vi "Process.vi"(8 "error in":errorcluster, 11 "LMT":refnum<class "LMT.lvclass">) -> (0 "error out":errorcluster, 3 "LMT out":refnum<class "LMT.lvclass">)   [LabVIEW 2017, in "LMT.lvclass"]
doc: "---------------------------------------------------------------\nJKI State Machine Objects™\nhttp://jki.net/state-machine-objects/\nCopyright (C) 2005-2015, JKI <info@jki.net>\nALL RIGHTS RESERVEDJKI State Machine Objects (SMO) 1.0.0.5\nJKI - JKI\nCopyright (c) 2016, JKI"
uses:
  LMT.lvclass
  D:/Program Files (x86)/National Instruments/LabVIEW 2017/vi.lib/JKI/JKI SMO/SMO/SMO.lvclass
  <vilib>/JKI/JKI SMO/SMO/Typedefs/SMOState --Enum.ctl
  <vilib>/JKI/JKI SMO/SMO/Typedefs/Parent Call--Enum.ctl
  <vilib>/JKI/JKI SMO/SMO/SMO.lvclass
panel:
  out "Dep2 GUID":string
  out "Dep1 GUID":string
  out "Dep2 Name":string
  out "Dep1 Name":string
  out "Dep2 State":T1
  out "Dep1 State":T1
  # "For instructions on how to use the JKI State Machine Objects, examples and video tutorials, visit:\nhttp://jki.net/state-machine-objects/\n\nJKI State Machine Objects™\nhttp://jki.net/state-machine-objects/\nCopyright (C) 2005-2015, JKI <info@jki.net>\nALL RIGHTS RESERVED"
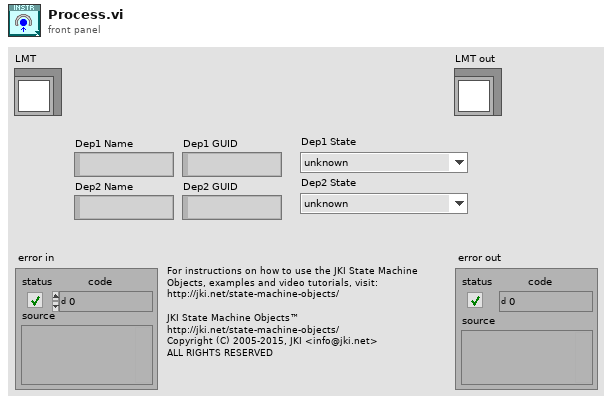
[diagram p1: front panel]
types:
  T1 = typedef "SMO.lvclass/SMOState --Enum.ctl" = enum16{"unknown", "Created", "Started", "Stopped"}
  T2 = typedef "SMO.lvclass/Parent Call--Enum.ctl" = enum16{"Allows parent to run", "Does not request parent to run"}
  T3 = enum32{"invalid app kind", "Development System", "Run Time System", "Student Edition", "Embedded LabVIEW", "Evaluation", "Custom"}
  T4 = enum32{"Invalid", "Standard", "Closed", "Hidden", "Minimized", "Maximized"}
  T5 = typedef "LMT.lvclass/Data.ctl" = string
  T6 = cluster{"Core":cluster{"Current VI Reference":refnum<vi>, "Close Panel on Exit?":bool, "error":errorcluster}, "Self Reference":refnum<class "LMT.lvclass">, "Your string data":string}
  T7 = cluster{"Current VI Reference":refnum<vi>, "Close Panel on Exit?":bool, "error":errorcluster}
  T8 = typedef "SMO.lvclass/Protected Events.ctl" = cluster{"StopProcesses":refnum<user-event>, "AbortProcesses":refnum<user-event>, "Config Changed":refnum<user-event>, "Dependency":refnum<user-event>}
  T9 = typedef "LMT.lvclass/ProtectedEvents--Cluster.ctl" = cluster{"API_Template":refnum<user-event>}
  T10 = typedef "LMT.lvclass/PrivateEvents--Cluster.ctl" = cluster{"AsyncMethod":refnum<user-event>}
  T11 = typedef "LMT.lvclass/Dependencies--Cluster.ctl" = cluster{"Dep1":refnum<class "SMO.lvclass">, "Dep2":refnum<class "SMO.lvclass">}
  T12 = typedef "SMO.lvclass/Public Events.ctl" = cluster{"Error":refnum<user-event>, "State":refnum<user-event>, "Reserve State":refnum<user-event>}
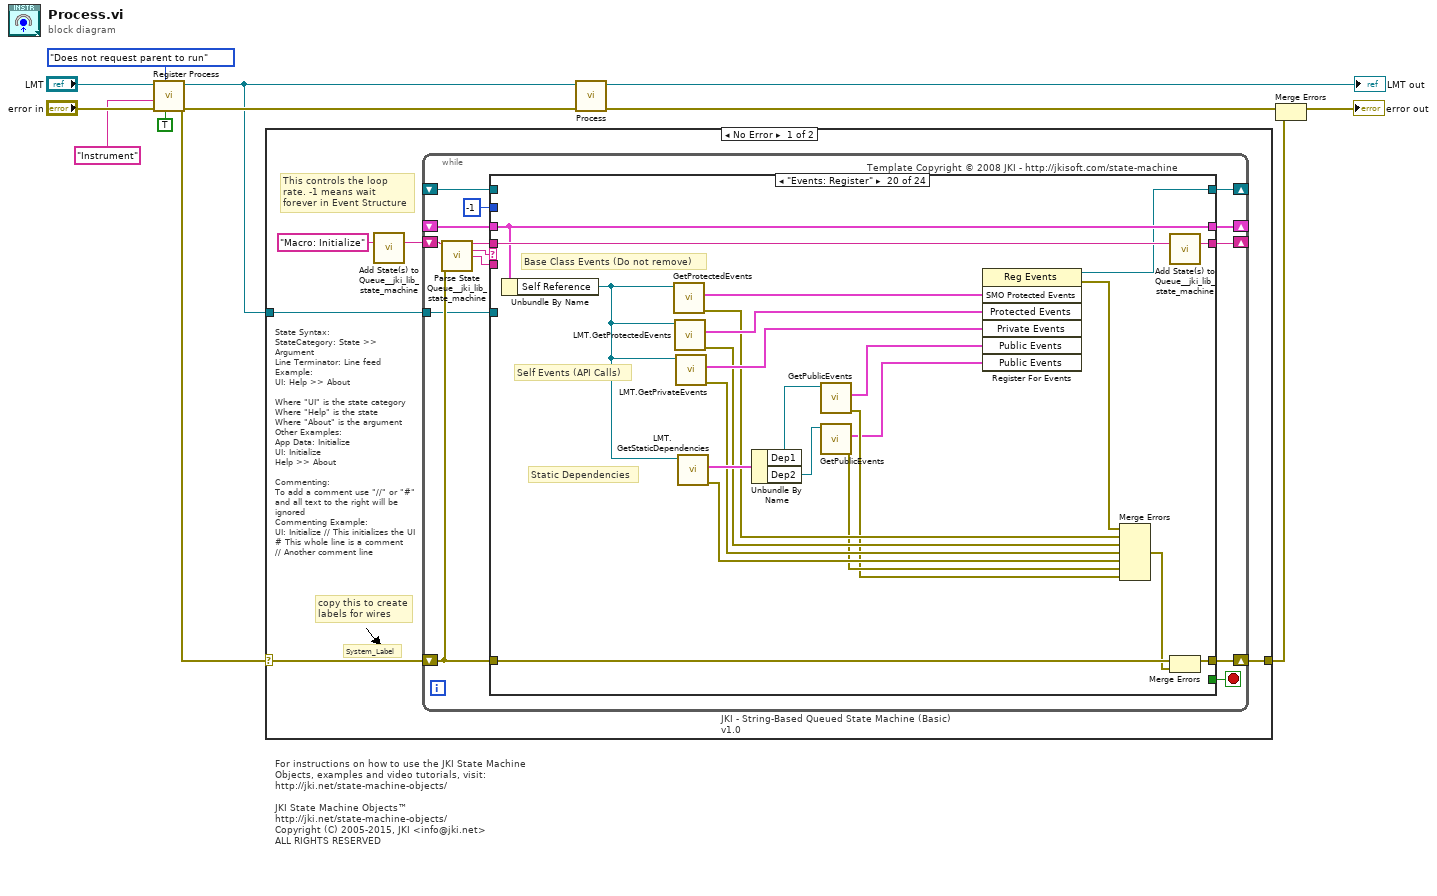
[diagram p0: block diagram]
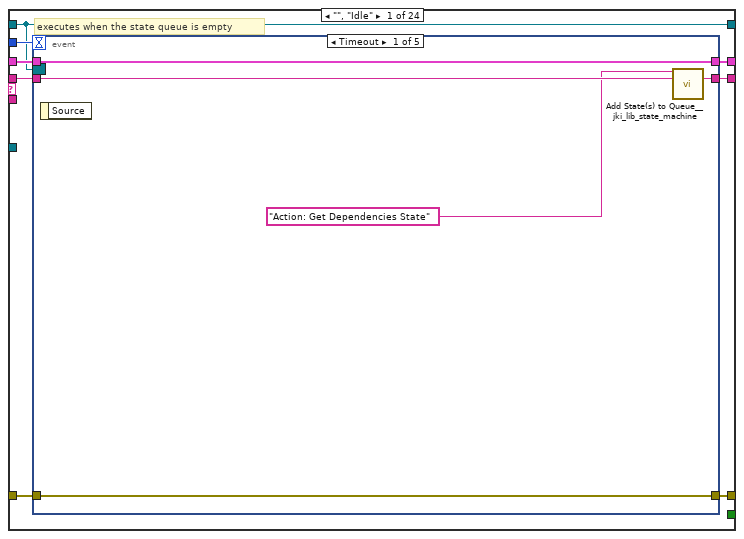
[diagram p2: hidden frame]
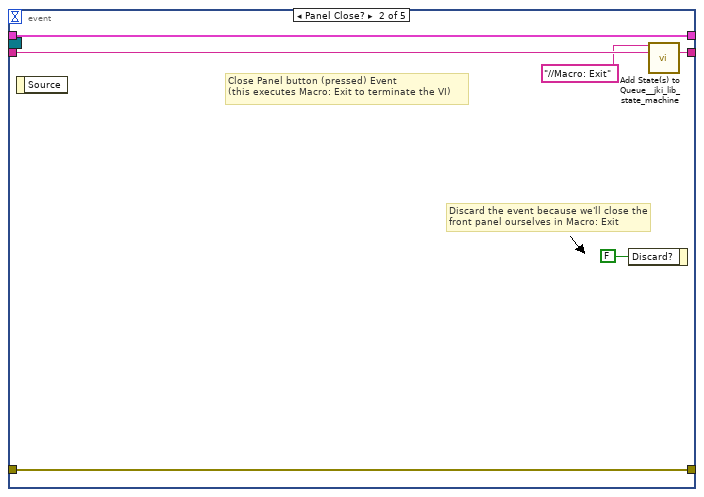
[diagram p3: hidden frame]
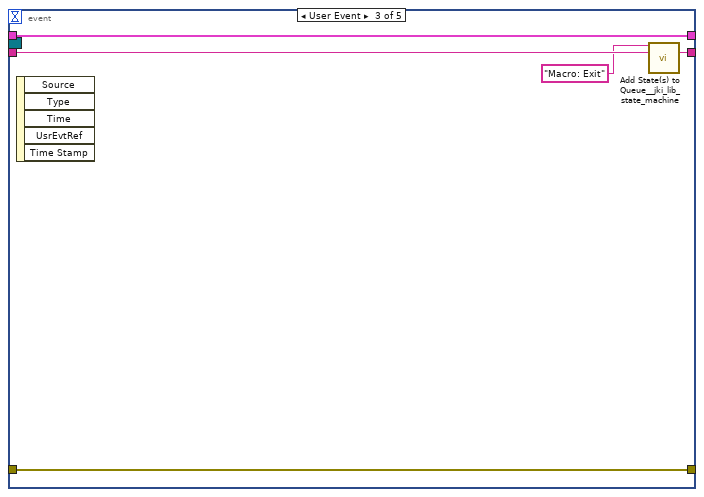
[diagram p4: hidden frame]
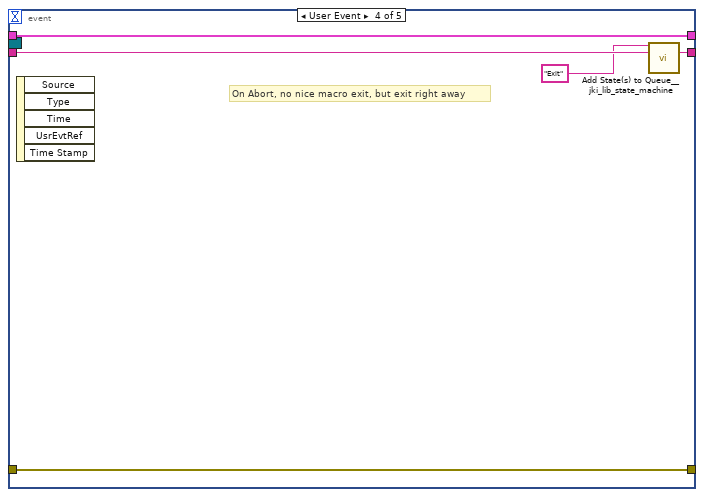
[diagram p5: hidden frame]
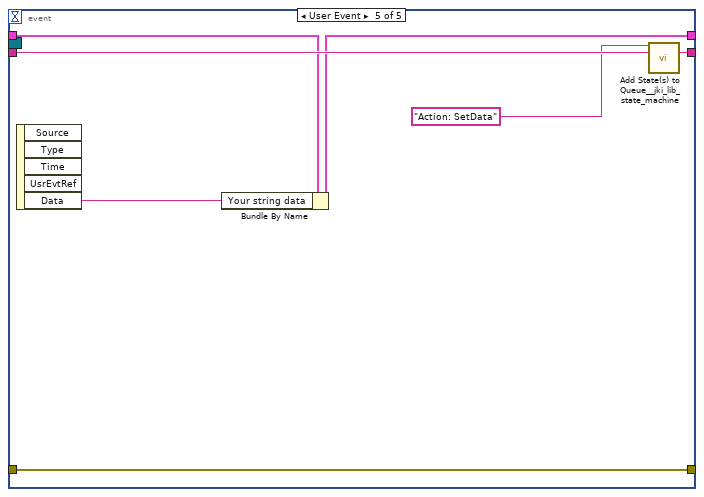
[diagram p6: hidden frame]
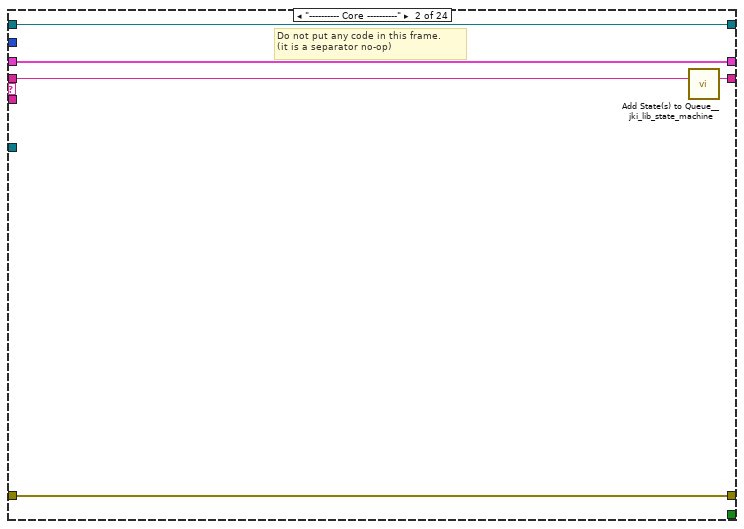
[diagram p7: hidden frame]
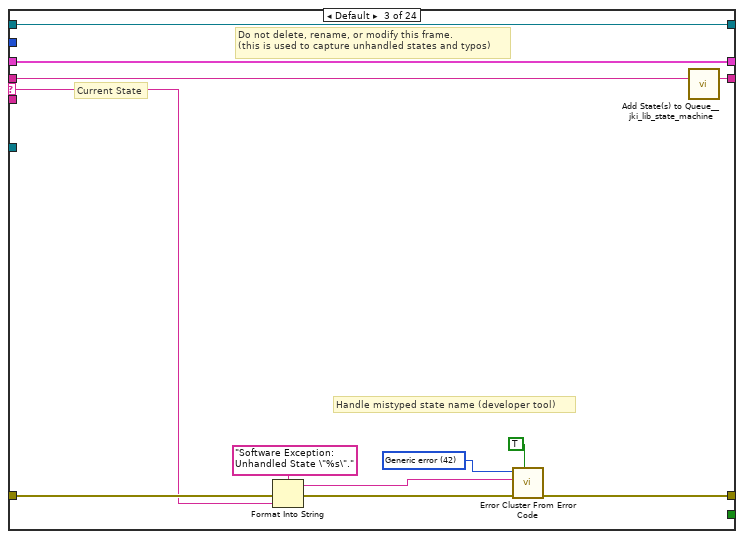
[diagram p8: hidden frame]
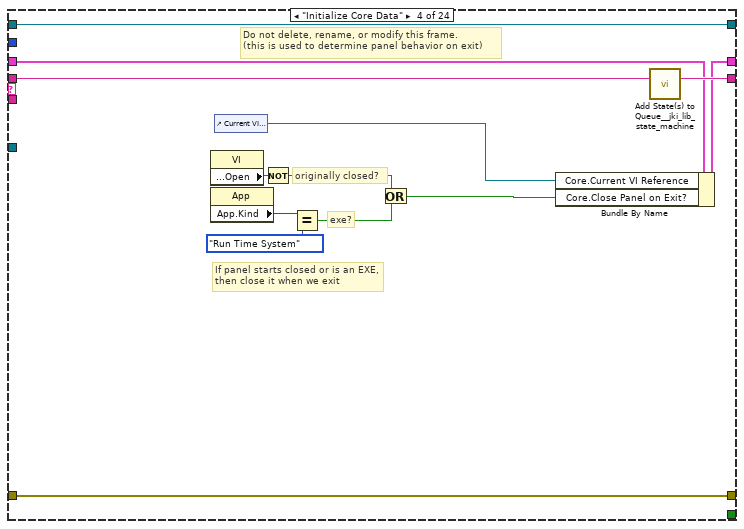
[diagram p9: hidden frame]
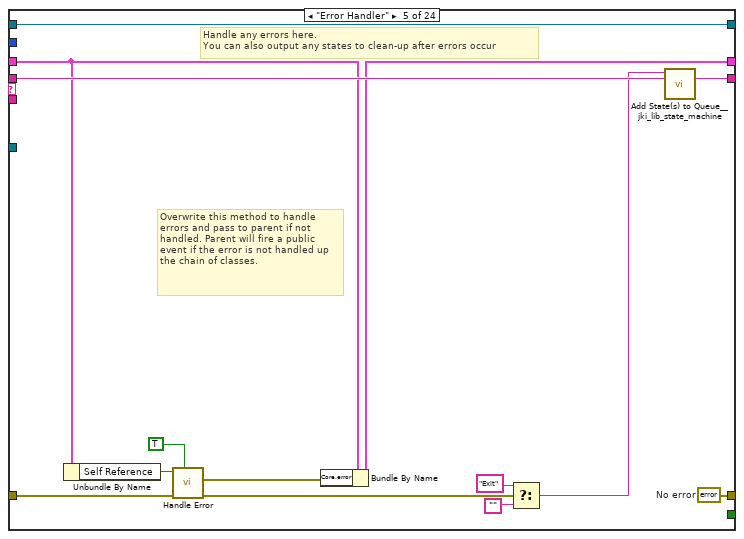
[diagram p10: hidden frame]
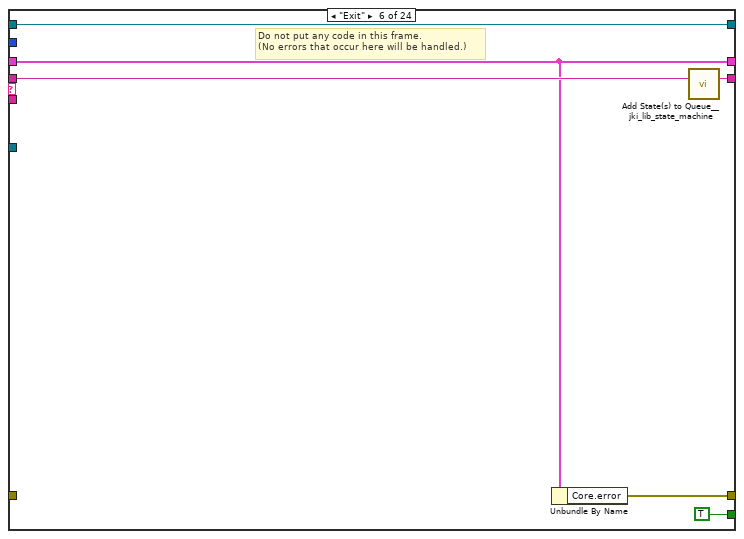
[diagram p11: hidden frame]
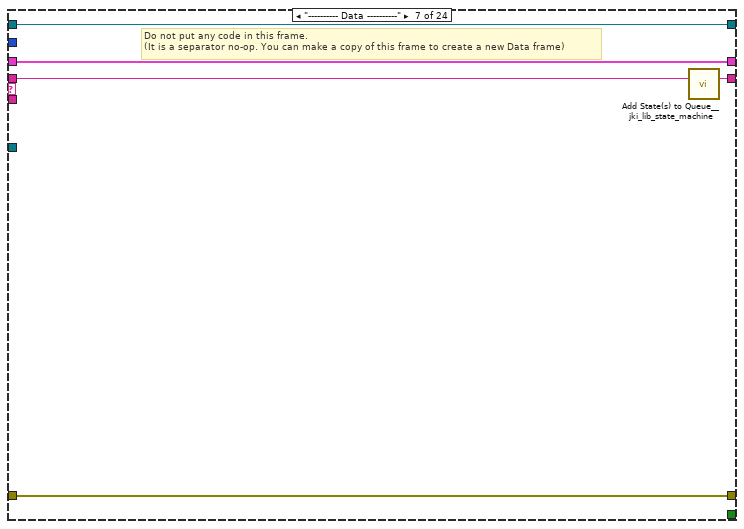
[diagram p12: hidden frame]
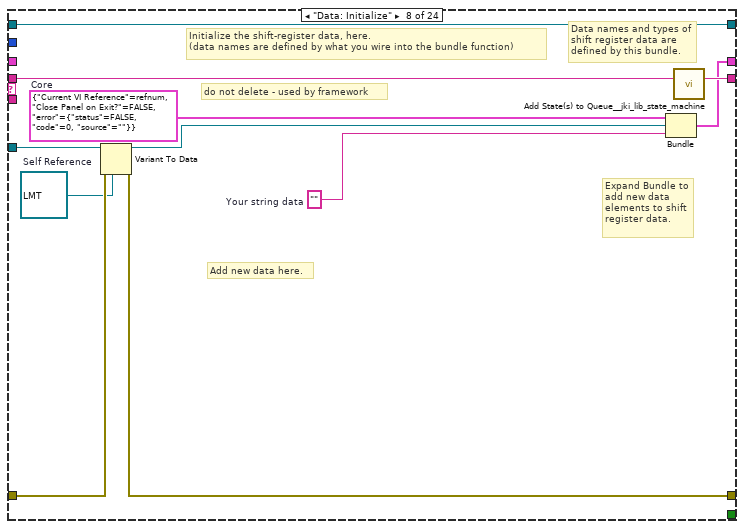
[diagram p13: hidden frame]
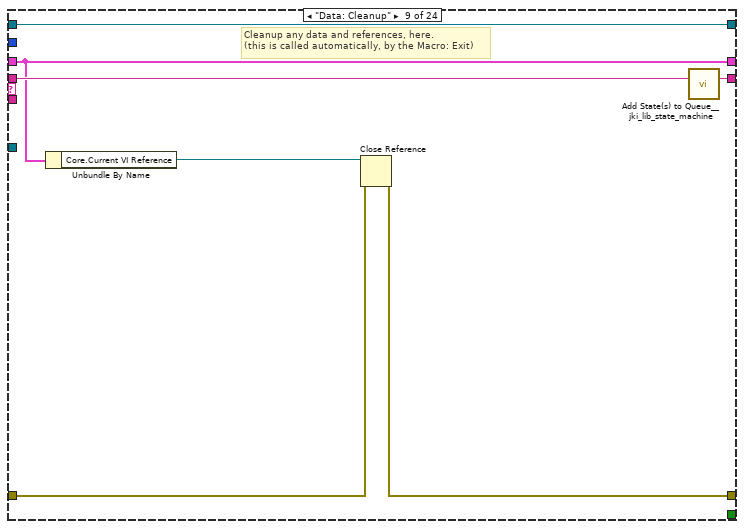
[diagram p14: hidden frame]
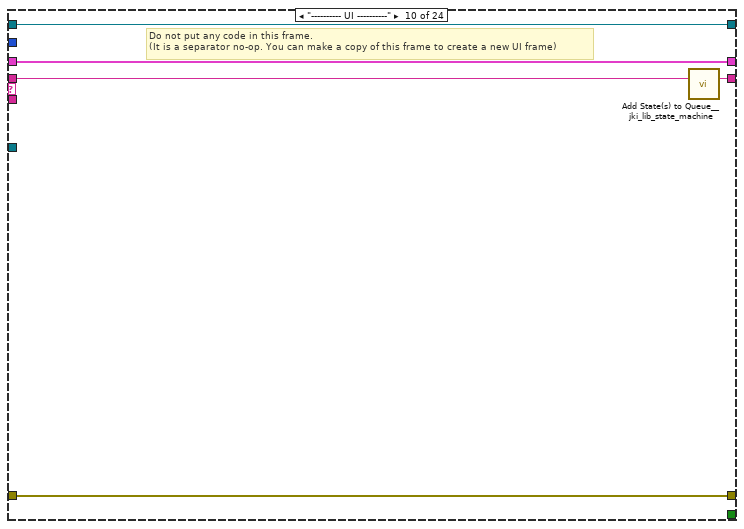
[diagram p15: hidden frame]
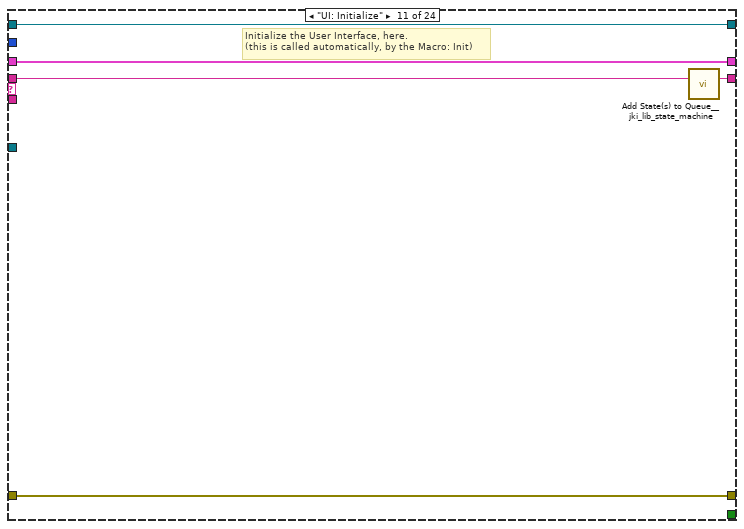
[diagram p16: hidden frame]
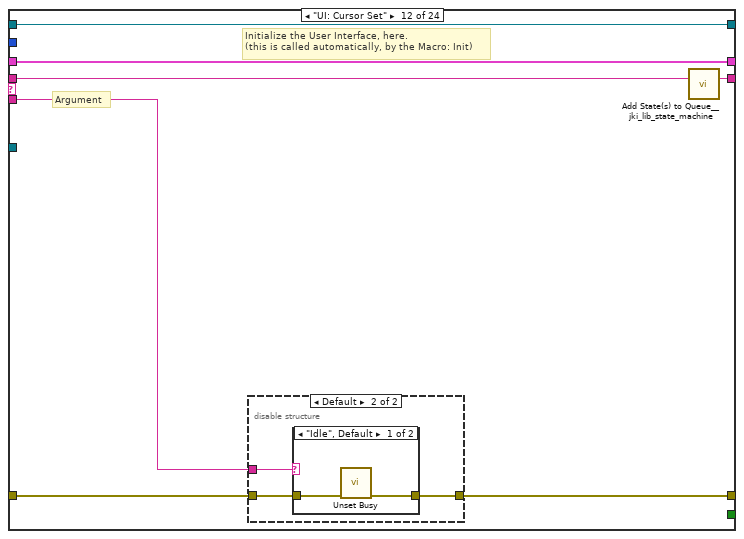
[diagram p17: hidden frame]
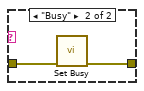
[diagram p19: hidden frame]
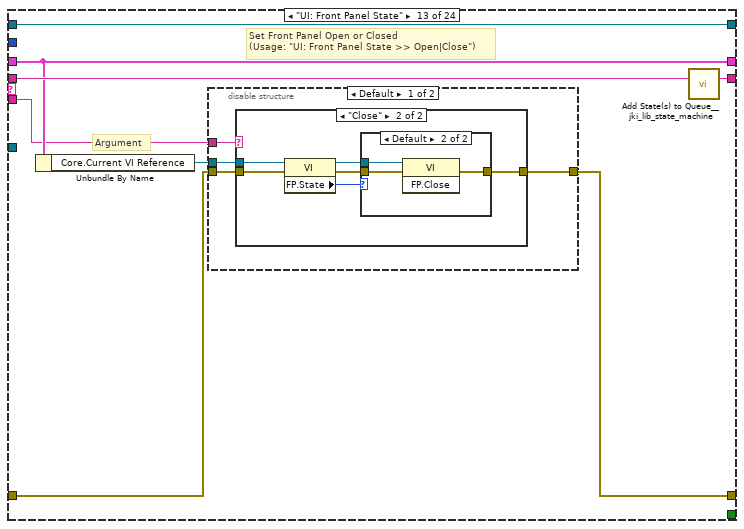
[diagram p20: hidden frame]
diagram:
  # "For instructions on how to use the JKI State Machine Objects, examples and video tutorials, visit:\nhttp://jki.net/state-machine-objects/\n\nJKI State Machine Objects™\nhttp://jki.net/state-machine-objects/\nCopyright (C) 2005-2015, JKI <info@jki.net>\nALL RIGHTS RESERVED"
  n1 = call <vilib>:"Register Process.vi"("Forces Self to Run (F)"=TRUE, "Parent Call"=Parent_Call--Enum."Does not request parent to run", "error in (no error)"="error in", "Process Name (optional)"="Instrument", "SMO"="LMT") -> ("error out"=w8:errorcluster, "SMO out"=w7:refnum<class "LMT.lvclass">)  [unwired: 5 in]
  n2 = case shown="No Error" w8 {
    selector: w8 -> [w13 w322]
    tunnel: w7 -> [w14 _]
    tunnel: [w12 w322] -> w4
    frame No Error {
      # "State Syntax:\nStateCategory: State >> Argument\nLine Terminator: Line feed\nExample:\nUI: Help >> About\n\nWhere \"UI\" is the state category\nWhere \"Help\" is the state\nWhere \"About\" is the argument\nOther Examples:\nApp Data: Initialize\nUI: Initialize\nHelp >> About\n\nCommenting:\nTo add a comment use \"//\" or \"#\" and all text to the right will be ignored\nCommenting Example:\nUI: Initialize // This initializes the UI\n# This whole line is a comment\n// Another comment line"
      # "copy this to create labels for wires"
      # "This controls the loop rate. -1 means wait forever in Event Structure"
      # "System_Label"
      n3 = call <vilib>:"Add State(s) to Queue__jki_lib_state_machine.vi"("State(s) in (\"\")"="Macro: Initialize") -> ("States Out"=w16:string)  [unwired: 14 in]
      n4 = while "JKI - String-Based Queued State Machine (Basic) v1.0" {
        shift-right: [w23] -> _
        shift-left: _ -> [w22]
        shift-right: [w26] -> w12
        shift-left: w13 -> [w20]
        shift-right: [w25] -> _
        shift-left: w16 -> [w27]
        tunnel: w14 -> [w19]
        shift-right: [w18] -> _
        shift-left: _ -> [w17]
        stop <- w24 stop-if-true
        # "Template Copyright © 2008 JKI - http://jkisoft.com/state-machine"
        n5 = call <vilib>:"Parse State Queue__jki_lib_state_machine.vi"("State Queue"=w27, "Error In (no error)"=w20) -> ("Remaining States"=w29:string, "Current State"=w30:string, "Arguments"=w28:string)  [unwired: 11 in]
        n6 = case shown="\"Events: Register\"" w30 {
          selector: w30 -> [_ _ w73 _ _ _ _ _ _ _ _ _ _ _ _ _ _ _ _ _ _ _ _ _]
          tunnel: w29 -> [w38 w71 w77 w96 w110 w116 w121 w132 w139 w144 w149 w156 w172 w204 w213 w227 w232 w243 w248 w271 w277 w282 w290 w318]
          tunnel: w28 -> [_ _ _ _ _ _ _ _ _ _ _ w150 w166 _ _ _ _ _ _ _ _ _ _ _]
          tunnel: w22 -> [w36 w68 w75 w87 w99 w112 w118 _ w134 w141 w147 w154 w168 w201 w209 w218 w229 w240 w245 w269 w275 w280 w287 w301]
          tunnel: [w35 w69 w79 w93 w101 w111 w119 w127 w135 w142 w146 w151 w169 w202 w211 w225 w230 w234 w246 w261 w273 w278 w283 w293] -> w26
          tunnel: w20 -> [w34 w69 w78 w93 w106 _ w119 w128 w136 w142 w146 w152 w170 w202 w211 w225 w230 w235 w246 w262 w273 w278 w284 w300]
          tunnel: [w37 w70 w76 w95 w109 w115 w120 w131 w138 w143 w148 w155 w171 w203 w212 w226 w231 w242 w247 w270 w276 w281 w289 w317] -> w25
          tunnel: [_ _ _ _ _ TRUE _ _ _ _ _ _ _ _ _ _ _ _ _ _ _ _ _ _] -> w24
          tunnel: [w33 w68 w75 w94 w98 w112 w118 w130 w134 w141 w147 w154 w168 w201 w209 w218 w229 w240 w245 w269 w275 w280 w287 w301] -> w23
          tunnel: -1 ("Timeout") -> [w32 _ _ _ _ _ _ _ _ _ _ _ _ _ _ _ _ _ _ _ _ _ _ _]
          tunnel: w19 -> [_ _ _ _ _ _ _ w125 _ _ _ _ _ _ _ _ _ _ _ _ _ _ _ _]
          tunnel: [w31 w67 w72 w84 w108 w113 w117 w123 w133 w140 w145 w153 w165 w200 w210 w219 w228 w241 w244 w268 w274 w279 w288 w316] -> w18
          tunnel: w17 -> [w31 w67 w72 w84 w108 w113 w117 w123 w133 w140 w145 w153 w165 w200 w210 w219 w228 w241 w244 _ w274 w279 w288 w316]
          frame "", "Idle" {
            # "executes when the state queue is empty"
            n7 = event shown="[0] Timeout" {
              selector: w31 -> [_ _ _ _ _]
              dyn-events: _ -> [_ _ _ _ _]
              timeout: w32 -> [_ _ _ _ _]
              tunnel: w38 -> [w43 w49 w54 w59 w66]
              tunnel: [w42 w48 w53 w58 w65] -> w37
              tunnel: w36 -> [w41 w46 w51 w56 w62]
              tunnel: [w40 w47 w52 w57 w64] -> w35
              tunnel: w34 -> [w40 w47 w52 w57 w64]
              tunnel: [w41 w46 w51 w56 w61] -> w33
              event Timeout {
                n8 = event-data() -> ()  [unwired: 1 in, 1 out]
                n9 = call <vilib>:"Add State(s) to Queue__jki_lib_state_machine.vi"("State(s) in Front (\"\")"="Action: Get Dependencies State", "State(s) in (\"\")"=w43) -> ("States Out"=w42:string)  [unwired: 13 in]
              }
              event Panel Close? {
                # "Discard the event because we'll close the front panel ourselves in Macro: Exit"
                # "Close Panel button (pressed) Event\n(this executes Macro: Exit to terminate the VI)"
                n10 = event-data() -> ()  [unwired: 1 in, 1 out]
                n11 = event-data("Discard?"=FALSE) -> ()  [unwired: 1 in, 1 out]
                n12 = call <vilib>:"Add State(s) to Queue__jki_lib_state_machine.vi"("State(s) in Front (\"\")"="//Macro: Exit", "State(s) in (\"\")"=w49) -> ("States Out"=w48:string)  [unwired: 13 in]
              }
              event User Event {
                n13 = event-data() -> ()  [unwired: 1 in, 5 out]
                n14 = call <vilib>:"Add State(s) to Queue__jki_lib_state_machine.vi"("State(s) in Front (\"\")"="Macro: Exit", "State(s) in (\"\")"=w54) -> ("States Out"=w53:string)  [unwired: 13 in]
              }
              event User Event {
                # "On Abort, no nice macro exit, but exit right away"
                n15 = event-data() -> ()  [unwired: 1 in, 5 out]
                n16 = call <vilib>:"Add State(s) to Queue__jki_lib_state_machine.vi"("State(s) in Front (\"\")"="Exit", "State(s) in (\"\")"=w59) -> ("States Out"=w58:string)  [unwired: 13 in]
              }
              event User Event {
                n17 = event-data() -> ("Data"=w63:T5)  [unwired: 1 in, 4 out]
                n18 = Bundle By Name(cluster=w62, "Your string data"=w63) -> (w61:T6)
                n19 = call <vilib>:"Add State(s) to Queue__jki_lib_state_machine.vi"("State(s) in Front (\"\")"="Action: SetData", "State(s) in (\"\")"=w66) -> ("States Out"=w65:string)  [unwired: 13 in]
              }
            }
          }
          frame "---------- Core ----------" {
            # "Do not put any code in this frame.\n(it is a separator no-op)"
            n20 = call <vilib>:"Add State(s) to Queue__jki_lib_state_machine.vi"("State(s) in (\"\")"=w71) -> ("States Out"=w70:string)  [unwired: 14 in]
          }
          frame Default {
            w82 = 42 items=["No error", "Argument error", "Memory is full", "Out of zone", "End of file", "File already open", "Generic file I/O error", "File not found", "File permission error", "Disk is full", "Duplicate path", "Too many files open", "System feature not enabled", "Resource file not found", "Cannot add resource", "Resource not found", "Image not found", "Image memory error", "Pen does not exist", "Config type invalid", "Config token not found", "Config parse error", "Config memory error", "Bad external code format", "Bad external code offset", "External code not present", "Null window", "Destroy window error", "Null menu", "Print aborted", "Bad print record", "Print driver error", "Windows error during printing", "Memory error during printing", "Print dialog error", "Generic print error", "Invalid device refnum", "Device not found", "Device parameter error", "Device unit error", "Cannot open device", "Device call aborted", "Generic error", "Cancelled by user", "Object ID too low", "Object ID too high", "Object not in heap", "Unknown heap", "Unknown object (invalid DefProc)", "Unknown object (DefProc not in table)", "Message out of range", "Invalid (null) method", "Unknown message", "Manager call not supported", "Bad address", "Network operation in progress", "Network operation timed out", "Connection is busy", "Network attribute not supported", "Network error", "Address in use", "System out of memory", "Connection aborted", "Connection refused", "Not connected", "Already connected", "Connection closed", "Initialization error (interapplication manager)", "Bad occurrence", "Wait on unbound occurrence handler", "Occurrence queue overflow", "Datalog type conflict", "Unused", "Unrecognized type (interapplication manager)", "Memory corrupt", "Failed to make temporary DLL", "Old CIN version", "Drag socket not found", "Failed to load drop-object", "Failed to register OLE object", "Failed to release OLE object", "Format specifier type mismatch", "Unknown format specifier", "Too few format specifiers", "Too many format specifiers", "Scan failed", "Newer CIN version", "Error converting to variant", "Runtime menu error", "Password tampered", "Variant attribute not found", "Incompatible variant data type", "Event data is not available", "Event Store is not present", "Occurrence is not found", "Event Queue is not created", "Event info is not available", "Refnum passed is NULL", "Error retrieving Class GUID", "Error retrieving CoClass GUID", "Error retrieving TypeLib GUID.", "Bad built application magic bytes.", "Specific driver is different from the specific driver associated with the Logical Name.", "There is no session opened to the class driver.", "Max Error", "MAX - Error with config objects", "MAX - Error loading configuration", "MAX - Group not supported"]
            # "Current State"
            # "Do not delete, rename, or modify this frame.\n(this is used to capture unhandled states and typos)"
            # "Handle mistyped state name (developer tool)"
            n21 = Format Into String(format string="Software Exception: Unhandled State \"%s\"." ("message"), error in=w78, w73) -> (resulting string=w81:string, error out=w80:errorcluster)  [unwired: 1 in]
            n22 = call <vilib>:"Error Cluster From Error Code.vi"("show call chain? (False)"=TRUE, "error in (no error)"=w80, "error message (\"\")"=w81, "error code (0)"=w82) -> ("error out"=w79:errorcluster)  [unwired: 5 in]
            n23 = call <vilib>:"Add State(s) to Queue__jki_lib_state_machine.vi"("State(s) in (\"\")"=w77) -> ("States Out"=w76:string)  [unwired: 14 in]
          }
          frame "Initialize Core Data" {
            # "Do not delete, rename, or modify this frame.\n(this is used to determine panel behavior on exit)"
            # "originally closed?"
            # "exe?"
            # "If panel starts closed or is an EXE, then close it when we exit"
            n24 = property class="VI"() -> ("Front Panel.Open"=w92:bool)  [unwired: 2 in, 2 out]
            n25 = property class="App"() -> ("App.Kind"=w91:T3)  [unwired: 2 in, 2 out]
            n26 = control-ref of="Current VI Reference"() -> (w85:refnum<vi>)
            n27 = Not(x=w92) -> (.not. x?=w89:bool)
            n28 = Equal?(x=w91, y=T3."Run Time System" ("Application:Kind")) -> (x = y?=w88:bool)
            n29 = Or(x=w89, y=w88) -> (x .or. y?=w86:bool)
            n30 = Bundle By Name(cluster=w87, "Core.Current VI Reference"=w85, "Core.Close Panel on Exit?"=w86) -> (w94:T6)
            n31 = call <vilib>:"Add State(s) to Queue__jki_lib_state_machine.vi"("State(s) in (\"\")"=w96) -> ("States Out"=w95:string)  [unwired: 14 in]
          }
          frame "Error Handler" {
            w101 = errorcluster {"status"=FALSE, "code"=0, "source"=""}  # No error
            # "Overwrite this method to handle errors and pass to parent if not handled. Parent will fire a public event if the error is not handled up the chain of classes."
            # "Handle any errors here.\nYou can also output any states to clean-up after errors occur"
            n32 = Unbundle By Name(w99) -> ("Self Reference"=w107:refnum<class "LMT.lvclass">)
            n33 = call-dynamic "Handle Error.vi"("Stop on Unhandled Error (T)"=TRUE, "error in"=w106, "SMO"=w107) -> ("handling error"=w102:errorcluster, "Unhandled error"=w100:errorcluster)  [unwired: 6 in, 1 out]
            n34 = Bundle By Name(cluster=w99, "Core.error"=w100) -> (w98:T6)
            n35 = Select(t="Exit", s=w102, f="") -> (s? t:f=w103:string)
            n36 = call <vilib>:"Add State(s) to Queue__jki_lib_state_machine.vi"("State(s) in Front (\"\")"=w103, "State(s) in (\"\")"=w110) -> ("States Out"=w109:string)  [unwired: 13 in]
          }
          frame "Exit" {
            # "Do not put any code in this frame.\n(No errors that occur here will be handled.)"
            n37 = Unbundle By Name(w112) -> ("Core.error"=w111:errorcluster)
            n38 = call <vilib>:"Add State(s) to Queue__jki_lib_state_machine.vi"("State(s) in (\"\")"=w116) -> ("States Out"=w115:string)  [unwired: 14 in]
          }
          frame "---------- Data ----------" {
            # "Do not put any code in this frame.\n(It is a separator no-op. You can make a copy of this frame to create a new Data frame)"
            n39 = call <vilib>:"Add State(s) to Queue__jki_lib_state_machine.vi"("State(s) in (\"\")"=w121) -> ("States Out"=w120:string)  [unwired: 14 in]
          }
          frame "Data: Initialize" {
            w122 = T7 {"Current VI Reference"=refnum, "Close Panel on Exit?"=FALSE, "error"={"status"=FALSE, "code"=0, "source"=""}}  # Core
            w126 = refnum<class "LMT.lvclass"> refnum  # Self Reference
            w129 = ""  # Your string data
            # "do not delete - used by framework"
            # "Expand Bundle to add new data elements to shift register data."
            # "Add new data here."
            # "Data names and types of shift register data are defined by this bundle."
            # "Initialize the shift-register data, here.\n(data names are defined by what you wire into the bundle function)"
            n40 = Variant To Data(error in=w128, type=w126, Variant=w125) -> (data=w124:refnum<class "LMT.lvclass">, error out=w127:errorcluster)
            n41 = Bundle("Core"=w122, "Self Reference"=w124, "Your string data"=w129) -> (w130:T6)  [unwired: 1 in]
            n42 = call <vilib>:"Add State(s) to Queue__jki_lib_state_machine.vi"("State(s) in (\"\")"=w132) -> ("States Out"=w131:string)  [unwired: 14 in]
          }
          frame "Data: Cleanup" {
            # "Cleanup any data and references, here.\n(this is called automatically, by the Macro: Exit)"
            n43 = Unbundle By Name(w134) -> ("Core.Current VI Reference"=w137:refnum<vi>)
            n44 = Close Reference(reference=w137, error in (no error)=w136) -> (error out=w135:errorcluster)
            n45 = call <vilib>:"Add State(s) to Queue__jki_lib_state_machine.vi"("State(s) in (\"\")"=w139) -> ("States Out"=w138:string)  [unwired: 14 in]
          }
          frame "---------- UI ----------" {
            # "Do not put any code in this frame.\n(It is a separator no-op. You can make a copy of this frame to create a new UI frame)"
            n46 = call <vilib>:"Add State(s) to Queue__jki_lib_state_machine.vi"("State(s) in (\"\")"=w144) -> ("States Out"=w143:string)  [unwired: 14 in]
          }
          frame "UI: Initialize" {
            # "Initialize the User Interface, here.\n(this is called automatically, by the Macro: Init)"
            n47 = call <vilib>:"Add State(s) to Queue__jki_lib_state_machine.vi"("State(s) in (\"\")"=w149) -> ("States Out"=w148:string)  [unwired: 14 in]
          }
          frame "UI: Cursor Set" {
            # "Argument"
            # "Initialize the User Interface, here.\n(this is called automatically, by the Macro: Init)"
            n48 = disable-structure shown="Default" {
              disable-tunnel: w152 -> [w157 w160]
              disable-tunnel: [w157 w159] -> w151
              disable-tunnel: w150 -> [_ w158]
              frame condition #0 {
              }
              frame condition #1 (active) {
                n49 = case shown="\"Idle\", Default" w158 {
                  tunnel: w160 -> [w162 w164]
                  tunnel: [w161 w163] -> w159
                  frame "Idle", Default {
                    n50 = call <vilib>:"Unset Busy.vi"("error in (no error)"=w162) -> ("error out"=w161:errorcluster)  [unwired: 10 in]
                  }
                  frame "Busy" {
                    n51 = call <vilib>:"Set Busy.vi"("error in (no error)"=w164) -> ("error out"=w163:errorcluster)  [unwired: 9 in, 1 out]
                  }
                }
              }
            }
            n52 = call <vilib>:"Add State(s) to Queue__jki_lib_state_machine.vi"("State(s) in (\"\")"=w156) -> ("States Out"=w155:string)  [unwired: 14 in]
          }
          frame "UI: Front Panel State" {
            # "Argument"
            # "Set Front Panel Open or Closed\n(Usage: \"UI: Front Panel State >> Open|Close\")"
            n53 = Unbundle By Name(w168) -> ("Core.Current VI Reference"=w167:refnum<vi>)
            n54 = disable-structure shown="Default" {
              disable-tunnel: w170 -> [w176 w199]
              disable-tunnel: [w175 w199] -> w169
              disable-tunnel: w167 -> [w174 _]
              disable-tunnel: w166 -> [w173 _]
              frame condition #0 (active) {
                n55 = case shown="\"Close\"" w173 {
                  tunnel: w176 -> [w180 w193]
                  tunnel: [w182 w194] -> w175
                  tunnel: w174 -> [w181 w191]
                  frame "Open", Default {
                    n56 = property class="VI"(reference=w181, error in=w180) -> (reference out=w178:refnum<vi>, error out=w179:errorcluster, "FP.State"=w177:T4)
                    n57 = case shown="\"Closed\"" w177 {
                      tunnel: [w185 w188] -> w182
                      tunnel: w179 -> [w184 w188]
                      tunnel: w178 -> [w183 _]
                      frame "Closed" {
                        n58 = invoke class="VI" method="FP.Open"(reference=w183, error in=w184, "Activate"=TRUE, "State"=T4."Standard") -> (error out=w185:errorcluster)  [unwired: 1 in, 4 out]
                      }
                      frame Default {
                      }
                    }
                  }
                  frame "Close" {
                    n59 = property class="VI"(reference=w191, error in=w193) -> (reference out=w190:refnum<vi>, error out=w192:errorcluster, "FP.State"=w189:T4)
                    n60 = case shown="Default" w189 {
                      tunnel: [w195 w198] -> w194
                      tunnel: w192 -> [w195 w197]
                      tunnel: w190 -> [_ w196]
                      frame "Invalid", "Closed" {
                      }
                      frame Default {
                        n61 = invoke class="VI" method="FP.Close"(reference=w196, error in=w197) -> (error out=w198:errorcluster)  [unwired: 1 in, 2 out]
                      }
                    }
                  }
                }
              }
              frame condition #1 {
              }
            }
            n62 = call <vilib>:"Add State(s) to Queue__jki_lib_state_machine.vi"("State(s) in (\"\")"=w172) -> ("States Out"=w171:string)  [unwired: 14 in]
          }
          frame "---------- Macro ----------" {
            # "Do not put any code in this frame.\n(It is a separator no-op. You can make a copy of this frame to create a new Macro frame)"
            n63 = call <vilib>:"Add State(s) to Queue__jki_lib_state_machine.vi"("State(s) in (\"\")"=w204) -> ("States Out"=w203:string)  [unwired: 14 in]
          }
          frame "Macro: Initialize" {
            w207 = "UI: Initialize\n//UI: Front Panel State >> Open"  # UI: Initialize //UI: Front Panel State >> Open
            # "Initialization Macro\n(This is called once, when the VI starts)"
            n64 = call <vilib>:"Add State(s) to Queue__jki_lib_state_machine.vi"("State(s) in Front (\"\")"="Data: Initialize\nInitialize Core Data\nEvents: Register\nAction: Get Dependencies State", "State(s) in (\"\")"="Process: Sync", "State(s) at Back (\"\")"=w207) -> ("States Out"=w206:string)  [unwired: 12 in]
            n65 = call <vilib>:"Add State(s) to Queue__jki_lib_state_machine.vi"("State(s) in Front (\"\")"=w206, "State(s) in (\"\")"=w213) -> ("States Out"=w212:string)  [unwired: 13 in]
          }
          frame "Macro: Exit" {
            # "Exit Macro\n(This is called once, when the VI exits)"
            n66 = Unbundle By Name(w218) -> ("Core.Close Panel on Exit?"=w224:bool)
            n67 = Select(t="UI: Front Panel State >> Close", s=w224, f="") -> (s? t:f=w221:string)
            n68 = call <vilib>:"Add State(s) to Queue__jki_lib_state_machine.vi"("State(s) in Front (\"\")"="Data: Cleanup\nEvents: Unregister", "State(s) in (\"\")"="Process: Sync", "State(s) at Back (\"\")"="Action: Get Dependencies State\nExit") -> ("States Out"=w215:string)  [unwired: 12 in]
            n69 = call <vilib>:"Add State(s) to Queue__jki_lib_state_machine.vi"("State(s) in (\"\")"=w221, "State(s) at Back (\"\")"=w215) -> ("States Out"=w220:string)  [unwired: 13 in]
            n70 = call <vilib>:"Add State(s) to Queue__jki_lib_state_machine.vi"("State(s) in Front (\"\")"=w220, "State(s) in (\"\")"=w227) -> ("States Out"=w226:string)  [unwired: 13 in]
          }
          frame "---------- Process ----------" {
            # "Template Separator\n(You can make a copy of, or modify, this frame)"
            n71 = call <vilib>:"Add State(s) to Queue__jki_lib_state_machine.vi"("State(s) in (\"\")"=w232) -> ("States Out"=w231:string)  [unwired: 14 in]
          }
          frame "Process: Sync" {
            n72 = Unbundle By Name(w240) -> ("Self Reference"=w236:refnum<class "LMT.lvclass">)
            n73 = call <vilib>:"WaitOnProcessSync.vi"("error in (no error)"=w235, "SMO"=w236) -> ("error out"=w234:errorcluster, "Don't run?"=w239:bool)  [unwired: 7 in, 1 out]
            n74 = Select(t="Data: Cleanup\nEvents: Unregister\nExit", s=w239, f="") -> (s? t:f=w233:string)
            n75 = call <vilib>:"Add State(s) to Queue__jki_lib_state_machine.vi"("State(s) in Front (\"\")"=w233, "State(s) in (\"\")"=w243) -> ("States Out"=w242:string)  [unwired: 13 in]
          }
          frame "---------- Events ----------" {
            # "Template Separator\n(You can make a copy of, or modify, this frame)"
            n76 = call <vilib>:"Add State(s) to Queue__jki_lib_state_machine.vi"("State(s) in (\"\")"=w248) -> ("States Out"=w247:string)  [unwired: 14 in]
          }
          frame "Events: Register" {
            # "Static Dependencies"
            # "Self Events (API Calls)"
            # "Base Class Events (Do not remove)"
            n77 = Unbundle By Name(w269) -> ("Self Reference"=w264:refnum<class "LMT.lvclass">)
            n78 = call <vilib>:"GetProtectedEvents.vi"("SMO"=w264) -> ("error out"=w259:errorcluster, "SMO Protected Events"=w267:T8)  [unwired: 8 in, 1 out]
            n79 = call "LMT.GetProtectedEvents.vi"("LMT"=w264) -> ("error out"=w258:errorcluster, "Protected Events"=w266:T9)  [unwired: 8 in, 1 out]
            n80 = call "LMT.GetPrivateEvents.vi"("LMT"=w264) -> ("error out"=w257:errorcluster, "Private Events"=w265:T10)  [unwired: 8 in, 1 out]
            n81 = call "LMT.GetStaticDependencies.vi"("LMT"=w264) -> ("error out"=w256:errorcluster, "Dependencies"=w263:T11)  [unwired: 8 in, 1 out]
            n82 = Unbundle By Name(w263) -> ("Dep1"=w254:refnum<class "SMO.lvclass">, "Dep2"=w253:refnum<class "SMO.lvclass">)
            n83 = call <vilib>:"GetPublicEvents.vi"("SMO"=w254) -> ("error out"=w251:errorcluster, "Public Events"=w250:T12)  [unwired: 8 in, 1 out]
            n84 = call <vilib>:"GetPublicEvents.vi"("SMO"=w253) -> ("error out"=w252:errorcluster, "Public Events"=w249:T12)  [unwired: 8 in, 1 out]
            n85 = register-events(w267, w266, w265, w250, w249) -> (reference out=w268:refnum<event-registration>, error out=w255:errorcluster)  [unwired: 2 in]
            n86 = Merge Errors(w255, w259, w258, w257, w256, w252, w251) -> (w260:errorcluster)
            n87 = call <vilib>:"Add State(s) to Queue__jki_lib_state_machine.vi"("State(s) in (\"\")"=w271) -> ("States Out"=w270:string)  [unwired: 14 in]
            n88 = Merge Errors(w262, w260) -> (w261:errorcluster)
          }
          frame "Events: Unregister" {
            n89 = Unregister For Events(event registration refnum=w274, error in=w273) -> (error out=w272:errorcluster)
            n90 = call <vilib>:"Clear Errors.vi"("error in (no error)"=w272) -> ()  [unwired: 5 in, 2 out]
            n91 = call <vilib>:"Add State(s) to Queue__jki_lib_state_machine.vi"("State(s) in (\"\")"=w277) -> ("States Out"=w276:string)  [unwired: 14 in]
          }
          frame "---------- Action ----------" {
            n92 = call <vilib>:"Add State(s) to Queue__jki_lib_state_machine.vi"("State(s) in (\"\")"=w282) -> ("States Out"=w281:string)  [unwired: 14 in]
          }
          frame "Action: SetData" {
            n93 = Unbundle By Name(w287) -> ("Self Reference"=w286:refnum<class "LMT.lvclass">, "Your string data"=w285:string)
            n94 = call-dynamic "LMT.SetData.vi"("error in (no error)"=w284, "Data"=w285, "LMT"=w286) -> ("error out"=w283:errorcluster)  [unwired: 7 in, 1 out]
            n95 = call <vilib>:"Add State(s) to Queue__jki_lib_state_machine.vi"("State(s) in (\"\")"=w290) -> ("States Out"=w289:string)  [unwired: 14 in]
          }
          frame "Action: Get Dependencies State" {
            n96 = Unbundle By Name(w301) -> ("Self Reference"=w315:refnum<class "LMT.lvclass">)
            n97 = call "LMT.GetStaticDependencies.vi"("error in (no error)"=w300, "LMT"=w315) -> ("error out"=w292:errorcluster, "Dependencies"=w314:T11)  [unwired: 7 in, 1 out]
            n98 = Unbundle By Name(w314) -> ("Dep1"=w311:refnum<class "SMO.lvclass">, "Dep2"=w308:refnum<class "SMO.lvclass">)
            n99 = Unbundle By Name(w292) -> ("code"=w291:i32)
            n100 = case shown="116" w291 {
              tunnel: [w319 w321] -> w293
              tunnel: w292 -> [w319 w320]
              frame Default {
              }
              frame 116 {
                # "Filter error 116 (flattening error when no deps)"
                n101 = call <vilib>:"Clear Errors.vi"("error in (no error)"=w320) -> ("error out"=w321:errorcluster)  [unwired: 5 in, 1 out]
              }
            }
            n102 = call <vilib>:"Get State.vi"("SMO"=w308) -> ("error out"=w296:errorcluster, "SMO State"=→"Dep2 State":T1, "SMO out"=w309:refnum<class "SMO.lvclass">)  [unwired: 8 in]
            n103 = call <vilib>:"Get State.vi"("SMO"=w311) -> ("error out"=w299:errorcluster, "SMO State"=→"Dep1 State":T1, "SMO out"=w313:refnum<class "SMO.lvclass">)  [unwired: 8 in]
            n104 = call <vilib>:"Get Name.vi"("error in (no error)"=w296, "SMO"=w309) -> ("error out"=w297:errorcluster, "Name"=→"Dep2 Name":string, "SMO out"=w310:refnum<class "SMO.lvclass">)  [unwired: 7 in]
            n105 = call <vilib>:"Get Name.vi"("error in (no error)"=w299, "SMO"=w313) -> ("error out"=w298:errorcluster, "Name"=→"Dep1 Name":string, "SMO out"=w312:refnum<class "SMO.lvclass">)  [unwired: 7 in]
            n106 = call <vilib>:"Get GUID.vi"("error in (no error)"=w297, "SMO"=w310) -> ("error out"=w294:errorcluster, "GUID"=→"Dep2 GUID":string)  [unwired: 7 in, 1 out]
            n107 = call <vilib>:"Get GUID.vi"("error in (no error)"=w298, "SMO"=w312) -> ("error out"=w295:errorcluster, "GUID"=→"Dep1 GUID":string)  [unwired: 7 in, 1 out]
            n108 = call <vilib>:"Clear Errors.vi"("error in (no error)"=w295) -> ()  [unwired: 5 in, 2 out]
            n109 = call <vilib>:"Clear Errors.vi"("error in (no error)"=w294) -> ()  [unwired: 5 in, 2 out]
            n110 = call <vilib>:"Add State(s) to Queue__jki_lib_state_machine.vi"("State(s) in (\"\")"=w318) -> ("States Out"=w317:string)  [unwired: 14 in]
          }
        }
      }
    }
    frame Error {
    }
  }
  n111 = call-parent "Process.vi"("error in"=w8, "SMO"=w7) -> ("error out"=w5:errorcluster, "SMO out"=→"LMT out":refnum<class "LMT.lvclass">)  [unwired: 8 in]
  n112 = Merge Errors(w5, w4) -> (→"error out":errorcluster)
